vi "ParseJSONObjectKey.vi"(8 "error in (no error)":errorcluster, 10 "offset past match":i32, 11 "JSON string":string) -> (0 "error out":errorcluster, 1 "key":string, 2 "offset out":i32, 3 "string copy":string)   [LabVIEW 2020]
uses:
  <vilib>/regexp/Match Regular Expression.xnode
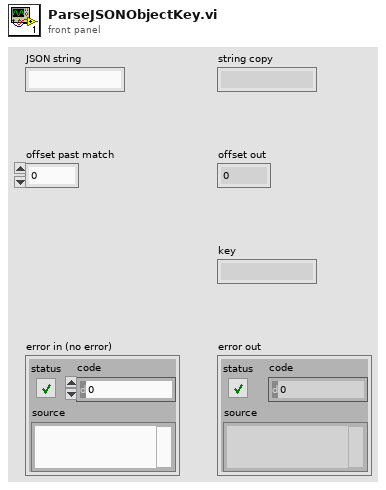
[diagram p1: front panel]
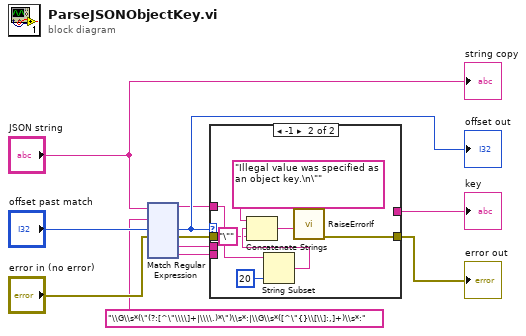
[diagram p0: block diagram]
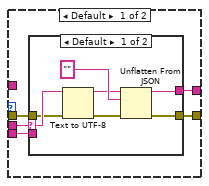
[diagram p2: hidden frame]
diagram:
  n1 = xnode "Match Regular Expression"("input string"="JSON string", "regular expression"="\\G\\s*(\"(?:[^\"\\\\]+|\\\\.)*\")\\s*:|\\G\\s*([^\"{}\\[\\]:,]+)\\s*:", "offset (0)"="offset past match", "error in"="error in (no error)") -> ("before match"=w1:string, "offset past match"=w3:i32, "error out"=w6:errorcluster, "submatch 1"=w8:string, "submatch 2"=w7:string)  [unwired: 2 in, 2 out]
  "offset out" <- w3
  n2 = case shown="-1" w3 {
    tunnel: w8 -> [w16 _]
    tunnel: w7 -> [w15 _]
    tunnel: w6 -> [w14 _]
    tunnel: [w13 w31] -> w5
    tunnel: [w12 _] -> w4
    tunnel: w1 -> [_ w29]
    frame Default {
      n3 = case shown="Default" w16 {
        selector: w16 -> [w22 _]
        tunnel: w15 -> [_ w25]
        tunnel: [w18 w25] -> w12
        tunnel: w14 -> [w20 w24]
        tunnel: [w17 w24] -> w13
        frame Default {
          n4 = Text to UTF-8(8:w20, 11:w22) -> (0:w19:errorcluster, 3:w21:string)  [unwired: 1 in]
          n5 = Unflatten From JSON(JSON string=w21, type and defaults="" ("whole match"), error in (no error)=w19) -> (value=w18:string, error out=w17:errorcluster)  [unwired: 4 in]
        }
        frame "" {
        }
      }
    }
    frame -1 {
      n6 = String Subset(string=w29, length (rest)=20 ("length (rest)")) -> (substring=w27:string)  [unwired: 1 in]
      n7 = Concatenate Strings("Illegal value was specified as an object key.\n\"" ("error message"), w27, "\"" ("string")) -> (w30:string)
      n8 = call "RaiseErrorIf.vi"("error message"=w30) -> ("error out"=w31:errorcluster)  [unwired: 10 in]
    }
  }
  "key" <- w4
  "error out" <- w5
  "string copy" <- "JSON string"
